vi "Configure.vi"(8 "error in (no error)":errorcluster, 10 "Args":string[](array[string]), 11 "Upgrade in":refnum<class "Upgrade.lvclass">) -> (0 "error out":errorcluster, 3 "Upgrade out":refnum<class "Upgrade.lvclass">)   [LabVIEW 2020, in "Upgrade.lvlib" / "Upgrade.lvclass"]
uses:
  Upgrade.lvclass
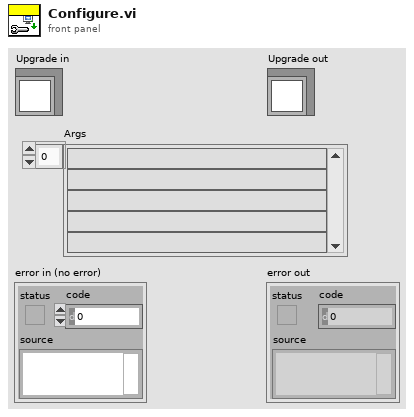
[diagram p1: front panel]
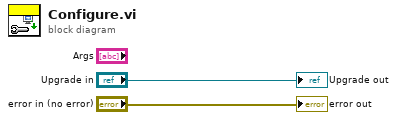
[diagram p0: block diagram]
diagram:
  "error out" <- "error in (no error)"
  "Upgrade out" <- "Upgrade in"
